vi "Labview ROS2 Bridge.vi"() -> ()   [LabVIEW 2021]
uses:
  <vilib>/RTI DDS Toolkit/Types/RTI DDS Advanced Writer Configuration.ctl
  <vilib>/RTI DDS Toolkit/Types/RTI DDS Advanced Reader Configuration.ctl
  <vilib>/RTI DDS Toolkit/VIs/AdvancedCreateReader_NumI32.vi
  <vilib>/RTI DDS Toolkit/VIs/AdvancedCreateWriter_NumI32.vi
  <vilib>/RTI DDS Toolkit/VIs/Write_NumI32.vi
  <vilib>/RTI DDS Toolkit/VIs/Read_NumI32.vi
  <vilib>/RTI DDS Toolkit/Library/LVDDS_library.lvlib
panel:
  out "RBF Weights":dbl[](array[numeric])
  in  "Advanced Reader Configuration 3":T1={"typeName"="std_msgs::msg::dds_::Int32_", "keyName"="", "domainParticipantQoSProfile"="", "dataReaderQoSProfile"="", "forceArrayMapping?"=FALSE, "forceExclusiveReader?"=FALSE, "forceRead? (only ExclusiveReader)"=FALSE, "forceUnboundedString?"=FALSE}
  out "Control Time (dt)":u32
  in  "Advanced Writer Configuration":T2={"typeName"="std_msgs::msg::dds_::Int32_", "keyName"="", "domainParticipantQoSProfile"="", "dataWriterQoSProfile"="", "forceArrayMapping?"=FALSE, "forceUnboundedString?"=FALSE}
  in  "stop":bool
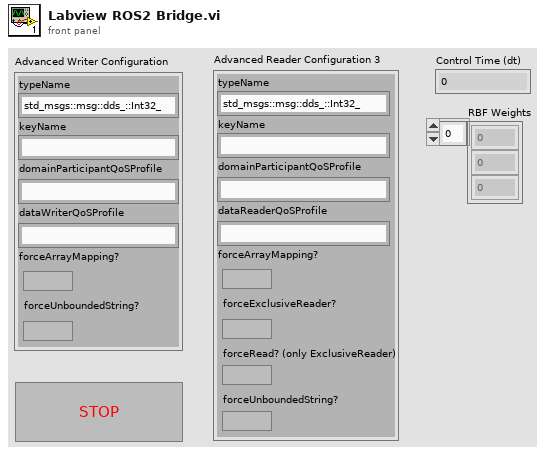
[diagram p1: front panel]
types:
  T1 = typedef "LVDDS_library.lvlib/RTI DDS Advanced Reader Configuration.ctl" = cluster{"typeName":string, "keyName":string, "domainParticipantQoSProfile":string, "dataReaderQoSProfile":string, "forceArrayMapping?":bool, "forceExclusiveReader?":bool, "forceRead? (only ExclusiveReader)":bool, "forceUnboundedString?":bool}
  T2 = typedef "LVDDS_library.lvlib/RTI DDS Advanced Writer Configuration.ctl" = cluster{"typeName":string, "keyName":string, "domainParticipantQoSProfile":string, "dataWriterQoSProfile":string, "forceArrayMapping?":bool, "forceUnboundedString?":bool}
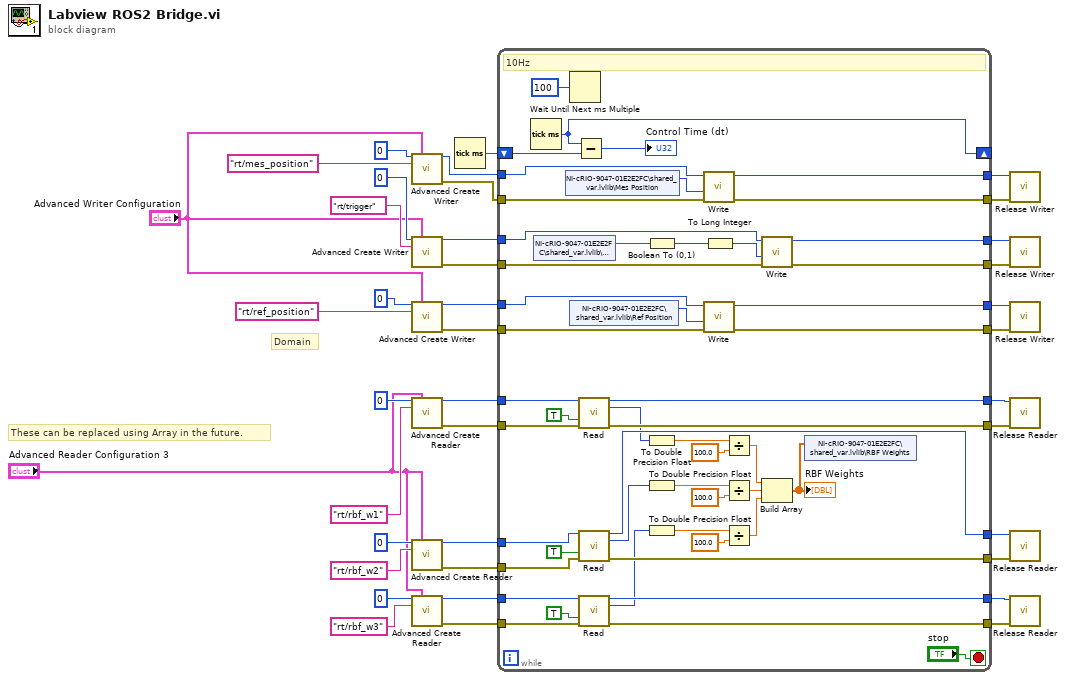
[diagram p0: block diagram]
diagram:
  # "These can be replaced using Array in the future."
  # "Domain"
  n1 = call-poly <vilib>:"Advanced Create Writer.vi"("Domain Id"=u32 0, "Advanced Writer Configuration"="Advanced Writer Configuration", "Topic Name"="rt/mes_position") -> ("DDS Object Ref"=w7:u64, "error out"=w8:errorcluster)  [unwired: 11 in]
  n2 = call-poly <vilib>:"Advanced Create Writer.vi"("Domain Id"=u32 0, "Advanced Writer Configuration"="Advanced Writer Configuration", "Topic Name"="rt/trigger") -> ("DDS Object Ref"=w37:u64, "error out"=w38:errorcluster)  [unwired: 11 in]
  n3 = call-poly <vilib>:"Advanced Create Writer.vi"("Domain Id"=u32 0, "Advanced Writer Configuration"="Advanced Writer Configuration", "Topic Name"="rt/ref_position") -> ("DDS Object Ref"=w10:u64, "error out"=w9:errorcluster)  [unwired: 11 in]
  n4 = call-poly <vilib>:"Advanced Create Reader.vi"("Domain Id"=u32 0, "Advanced Reader Configuration"="Advanced Reader Configuration 3", "Topic Name"="rt/rbf_w1") -> ("DDS Object Ref"=w18:u64, "error out"=w19:errorcluster)  [unwired: 11 in]
  n5 = call-poly <vilib>:"Advanced Create Reader.vi"("Domain Id"=u32 0, "Advanced Reader Configuration"="Advanced Reader Configuration 3", "Topic Name"="rt/rbf_w2") -> ("DDS Object Ref"=w25:u64, "error out"=w24:errorcluster)  [unwired: 11 in]
  n6 = call-poly <vilib>:"Advanced Create Reader.vi"("Domain Id"=u32 0, "Advanced Reader Configuration"="Advanced Reader Configuration 3", "Topic Name"="rt/rbf_w3") -> ("DDS Object Ref"=w31:u64, "error out"=w32:errorcluster)  [unwired: 11 in]
  n7 = Tick Count (ms)() -> (millisecond timer value=w28:u32)
  n8 = while {
    tunnel: w37 -> [w88]
    tunnel: [w87] -> w36
    tunnel: w38 -> [w89]
    tunnel: [w86] -> w35
    tunnel: w32 -> [w85]
    tunnel: [w82] -> w29
    tunnel: w31 -> [w84]
    tunnel: [w83] -> w30
    tunnel: w24 -> [w67]
    tunnel: [w70] -> w27
    tunnel: w25 -> [w68]
    tunnel: [w69] -> w26
    tunnel: w19 -> [w66]
    tunnel: [w63] -> w16
    tunnel: w18 -> [w65]
    tunnel: [w64] -> w17
    shift-right: [w51] -> _
    shift-left: w28 -> [w76]
    tunnel: w10 -> [w47]
    tunnel: [w48] -> w11
    tunnel: w9 -> [w46]
    tunnel: [w49] -> w12
    tunnel: w7 -> [w44]
    tunnel: [w43] -> w6
    tunnel: w8 -> [w45]
    tunnel: [w42] -> w5
    stop <- "stop" stop-if-true
    # "10Hz"
    n9 = Tick Count (ms)() -> (millisecond timer value=w51:u32)
    n10 = shared-variable "NI-cRIO-9047-01E2E2FC\\shared_var.lvlib\\Trigger"() -> (w80:bool)  [unwired: 1 in, 1 out]
    n11 = shared-variable "NI-cRIO-9047-01E2E2FC\\shared_var.lvlib\\Mes Position"() -> (w40:i32)  [unwired: 1 in, 1 out]
    n12 = Wait Until Next ms Multiple(millisecond multiple=u32 100) -> ()  [unwired: 1 out]
    n13 = shared-variable "NI-cRIO-9047-01E2E2FC\\shared_var.lvlib\\Ref Position"() -> (w41:i32)  [unwired: 1 in, 1 out]
    n14 = Subtract(x=w51, y=w76) -> (x-y=→"Control Time (dt)":u32)
    n15 = call-poly <vilib>:"Read.vi"("DDS Object Ref in"=w65, "Only New Samples"=TRUE, "error in (no error)"=w66) -> ("DDS Object Ref out"=w64:u64, "Data"=w58:i32, "error out"=w63:errorcluster)  [unwired: 8 in, 2 out]
    n16 = call-poly <vilib>:"Read.vi"("DDS Object Ref in"=w68, "Only New Samples"=TRUE, "error in (no error)"=w67) -> ("DDS Object Ref out"=w69:u64, "Data"=w59:i32, "error out"=w70:errorcluster)  [unwired: 8 in, 2 out]
    n17 = call-poly <vilib>:"Read.vi"("DDS Object Ref in"=w84, "Only New Samples"=TRUE, "error in (no error)"=w85) -> ("DDS Object Ref out"=w83:u64, "Data"=w57:i32, "error out"=w82:errorcluster)  [unwired: 8 in, 2 out]
    n18 = Boolean To (0,1)(Boolean=w80) -> (0, 1=w79:i16)
    n19 = To Double Precision Float(number=w58) -> (double precision float=w61:dbl)
    n20 = To Double Precision Float(number=w59) -> (double precision float=w72:dbl)
    n21 = To Double Precision Float(number=w57) -> (double precision float=w75:dbl)
    n22 = call-poly <vilib>:"Write.vi"("error in (no error)"=w45, "Data"=w40, "DDS Object Ref in"=w44) -> ("error out"=w42:errorcluster, "DDS Object Ref out"=w43:u64)  [unwired: 7 in]
    n23 = call-poly <vilib>:"Write.vi"("error in (no error)"=w46, "Data"=w41, "DDS Object Ref in"=w47) -> ("error out"=w49:errorcluster, "DDS Object Ref out"=w48:u64)  [unwired: 7 in]
    n24 = To Long Integer(number=w79) -> (32bit integer=w78:i32)
    n25 = Divide(x=w61, y=100.0) -> (x/y=w56:dbl)
    n26 = Divide(x=w72, y=100.0) -> (x/y=w55:dbl)
    n27 = Divide(x=w75, y=100.0) -> (x/y=w54:dbl)
    n28 = call-poly <vilib>:"Write.vi"("error in (no error)"=w89, "Data"=w78, "DDS Object Ref in"=w88) -> ("error out"=w86:errorcluster, "DDS Object Ref out"=w87:u64)  [unwired: 7 in]
    n29 = Build Array(w56, w55, w54) -> (w53:dbl[])
    "RBF Weights" <- w53
    n30 = shared-variable "NI-cRIO-9047-01E2E2FC\\shared_var.lvlib\\RBF Weights"(w53) -> ()  [unwired: 1 in, 1 out]
  }
  n31 = call <vilib>:"Release Writer.vi"("error in (no error)"=w5, "DDS Object Ref"=w6) -> ()  [unwired: 9 in, 1 out]
  n32 = call <vilib>:"Release Writer.vi"("error in (no error)"=w35, "DDS Object Ref"=w36) -> ()  [unwired: 9 in, 1 out]
  n33 = call <vilib>:"Release Writer.vi"("error in (no error)"=w12, "DDS Object Ref"=w11) -> ()  [unwired: 9 in, 1 out]
  n34 = call <vilib>:"Release Reader.vi"("error in (no error)"=w16, "DDS Object Ref"=w17) -> ()  [unwired: 9 in, 1 out]
  n35 = call <vilib>:"Release Reader.vi"("error in (no error)"=w27, "DDS Object Ref"=w26) -> ()  [unwired: 9 in, 1 out]
  n36 = call <vilib>:"Release Reader.vi"("error in (no error)"=w29, "DDS Object Ref"=w30) -> ()  [unwired: 9 in, 1 out]
